vi "Adding camera trigger to counter task_final.vi"() -> ()   [LabVIEW 2020]
uses:
  <vilib>/DAQmx/write.llb/DAQmx Write (Analog 1D DBL 1Chan NSamp).vi
  <vilib>/DAQmx/create/channels.llb/DAQmx Create Channel (AO-Voltage-Basic).vi
  <vilib>/Analysis/polynomials.llb/Polynomial Plot (Range).vi
  <vilib>/Utility/file.llb/Read Delimited Spreadsheet (DBL).vi
  <vilib>/DAQmx/configure/timing.llb/DAQmx Timing (Sample Clock).vi
  <vilib>/DAQmx/miscellaneous.llb/DAQmx Fill In Error Info.vi
  <vilib>/DAQmx/create/channels.llb/DAQmx Create Channel (CO-Pulse Generation-Frequency).vi
  <vilib>/DAQmx/configure/timing.llb/DAQmx Timing (Implicit).vi
  <vilib>/DAQmx/create/channels.llb/DAQmx Create Channel (CO-Pulse Generation-Ticks).vi
  <resource>/objmgr/daqmx.rc
  <vilib>/Analysis/NI_AALPro.lvlib
panel:
  in  "How many datapoints?":i32=1025
  in  "File to read":path=path "C:/Users/Hannah/Downloads/newcalibration_voice coil input_25msflyback.txt"
  in  "P(x)":dbl[](array[numeric])=[-0.285, 0.654, -0.163]
  out "polynomial plot":cluster{dbl[], "P(A)":dbl[]}(graph)
  out "# Samples written per channel":u32=1000
  out "actual frequency":dbl=1000.0
  in  "stop":bool
  out "Signal input to voice coil (blue)":dbl[](graph)
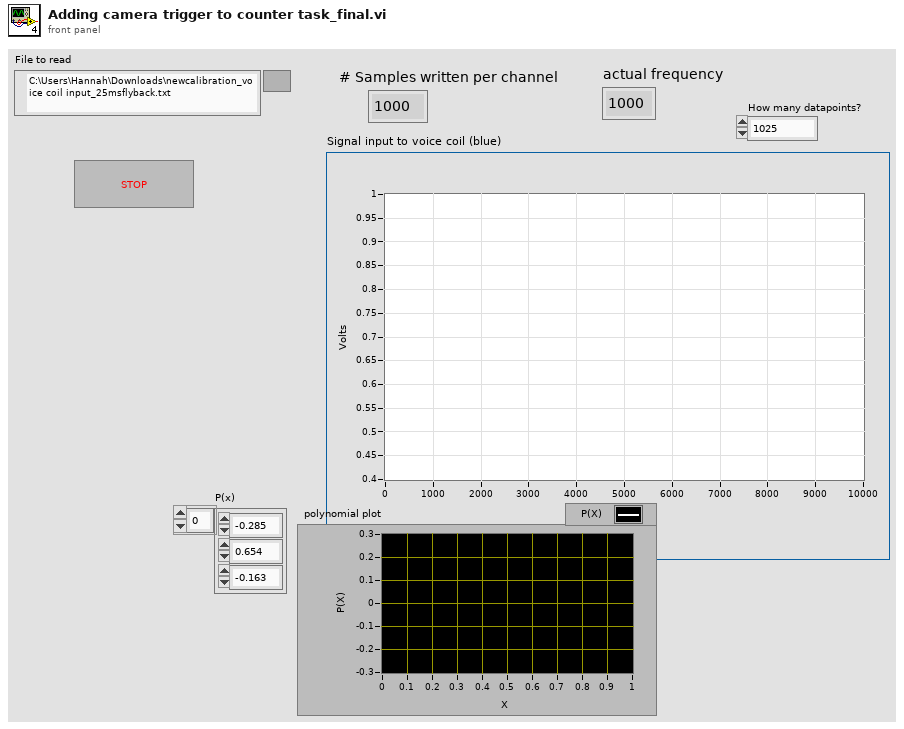
[diagram p1: front panel]
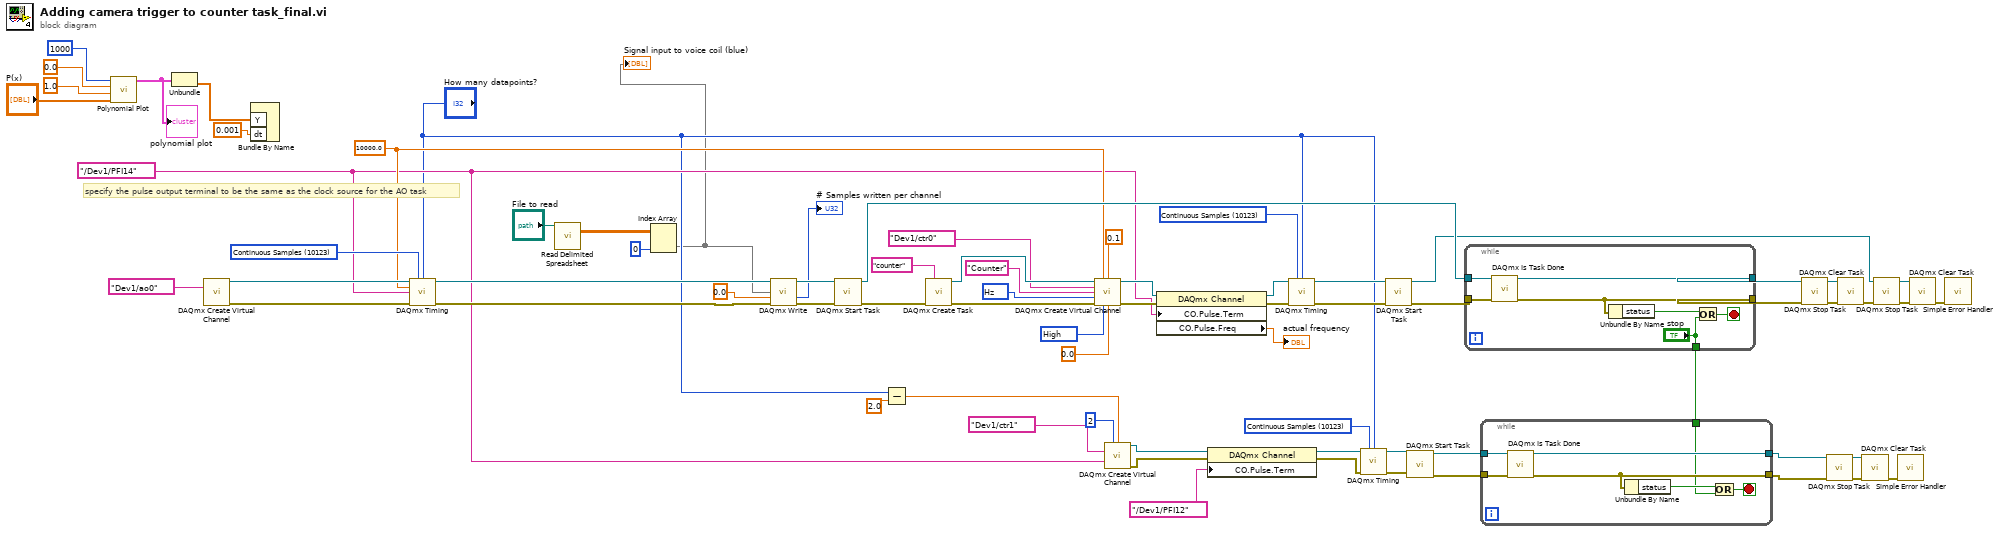
[diagram p0: block diagram]
diagram:
  w10 = 10123 items=["Finite Samples"=10178, "Continuous Samples"=10123, "Hardware Timed Single Point"=12522] ("sample mode")
  w43 = 10192 items=["High"=10192, "Low"=10214] ("idle state")
  w44 = 10373 items=["Hz"=10373] ("units")
  w7 = tag "/Dev1/PFI14" ("CO.Pulse.Term")
  w24 = 10123 items=["Finite Samples"=10178, "Continuous Samples"=10123, "Hardware Timed Single Point"=12522] ("sample mode")
  w20 = 10000.0 ("rate")
  w70 = 10123 items=["Finite Samples"=10178, "Continuous Samples"=10123, "Hardware Timed Single Point"=12522] ("sample mode")
  # "specify the pulse output terminal to be the same as the clock source for the AO task"
  n1 = call-poly <vilib>:"Polynomial Plot.vi"("P(x)"="P(x)", "end"=1.0, "start"=0.0, "samples"=1000) -> ("polynomial plot"=w38:cluster{"Ramp Pattern":dbl[], "P(A)":dbl[]})  [unwired: 6 in, 1 out]
  "polynomial plot" <- w38
  n2 = Unbundle(w38) -> ("P(A)"=w2:dbl[])  [unwired: 1 out]
  n3 = call-poly <vilib>:"DAQmx Create Virtual Channel.vi"("physical channels"=tag "Dev1/ao0") -> ("task out"=w72:refnum<k21>, "error out"=w71:errorcluster)  [unwired: 13 in]
  n4 = Bundle By Name("Y"=w2, "dt"=0.001) -> ()  [unwired: 1 in, 1 out]
  n5 = call-poly <vilib>:"DAQmx Timing.vi"("task/channels in"=w72, "sample mode"=w70, "samples per channel"="How many datapoints?", "rate"=w20, "source"=w7, "error in"=w71) -> ("task out"=w28:refnum<k21>, "error out"=w27:errorcluster)  [unwired: 8 in]
  n6 = call-poly <vilib>:"Read Delimited Spreadsheet.vi"("file path (dialog if empty)"="File to read") -> ("all rows"=w32:dbl[][])  [unwired: 9 in, 5 out]
  n7 = Index Array(array=w32, index (col)=0 ("disabled index (col)")) -> (element=w1:dbl[])  [unwired: 1 in]
  "Signal input to voice coil (blue)" <- w1
  n8 = call-poly <vilib>:"DAQmx Write.vi"("task/channels in"=w28, "data"=w1, "timeout"=0.0, "error in"=w27) -> ("task out"=w49:refnum<k21>, "number of samples written per channel"=→"# Samples written per channel":u32, "error out"=w48:errorcluster)  [unwired: 9 in]
  n9 = call <vilib>:"DAQmx Start Task.vi"("task/channels in"=w49, "error in"=w48) -> ("task out"=w42:refnum<k21>, "error out"=w41:errorcluster)  [unwired: 12 in]
  n10 = Subtract(x="How many datapoints?", y=2.0) -> (x-y=w5:dbl)
  n11 = call <vilib>:"DAQmx Create Task.vi"("new task name"="counter", "error in"=w41) -> ("task out"=w65:refnum<k21>, "error out"=w63:errorcluster)  [unwired: 12 in]
  n12 = call-poly <vilib>:"DAQmx Create Virtual Channel.vi"("task in"=w65, "frequency"=w20, "duty cycle"=0.1, "counter"=tag "Dev1/ctr0", "name to assign"="Counter", "units"=w44, "error in"=w63, "idle state"=w43, "initial delay"=0.0) -> ("task out"=w62:refnum<k21>, "error out"=w61:errorcluster)  [unwired: 5 in]
  n13 = call-poly <vilib>:"DAQmx Create Virtual Channel.vi"("high ticks"=u32 2, "low ticks"=w5, "counter"=tag "Dev1/ctr1", "source of ticks"=w7) -> ("task out"=w19:refnum<k21>, "error out"=w18:errorcluster)  [unwired: 10 in]
  n14 = property class="DAQmx Channel"(reference=w62, error in=w61, "CO.Pulse.Term"=w7) -> (reference out=w58:refnum<k21>, error out=w59:errorcluster, "CO.Pulse.Freq"=→"actual frequency":dbl)
  n15 = property class="DAQmx Channel"(reference=w19, error in=w18, "CO.Pulse.Term"=tag "/Dev1/PFI12") -> (reference out=w12:refnum<k21>, error out=w11:errorcluster)
  n16 = call-poly <vilib>:"DAQmx Timing.vi"("task/channels in"=w58, "sample mode"=w24, "samples per channel"="How many datapoints?", "error in"=w59) -> ("task out"=w68:refnum<k21>, "error out"=w67:errorcluster)  [unwired: 10 in]
  n17 = call-poly <vilib>:"DAQmx Timing.vi"("task/channels in"=w12, "sample mode"=w10, "samples per channel"="How many datapoints?", "error in"=w11) -> ("task out"=w9:refnum<k21>, "error out"=w8:errorcluster)  [unwired: 10 in]
  n18 = call <vilib>:"DAQmx Start Task.vi"("task/channels in"=w68, "error in"=w67) -> ("task out"=w30:refnum<k21>, "error out"=w50:errorcluster)  [unwired: 12 in]
  n19 = call <vilib>:"DAQmx Start Task.vi"("task/channels in"=w9, "error in"=w8) -> ("task out"=w16:refnum<k21>, "error out"=w15:errorcluster)  [unwired: 12 in]
  n20 = while {
    tunnel: w42 -> [w80]
    tunnel: w50 -> [w79]
    tunnel: [w78] -> w54
    tunnel: [w77] -> w55
    tunnel: ["stop"] -> w3
    stop <- w75 stop-if-true
    n21 = call <vilib>:"DAQmx Is Task Done.vi"("task/channels in"=w80, "error in"=w79) -> ("task out"=w78:refnum<k21>, "error out"=w77:errorcluster)  [unwired: 11 in, 1 out]
    n22 = Unbundle By Name(w77) -> ("status"=w76:bool)
    n23 = Or(x=w76, y="stop") -> (x .or. y?=w75:bool)
  }
  n24 = while {
    tunnel: w16 -> [w87]
    tunnel: w15 -> [w86]
    tunnel: [w85] -> w14
    tunnel: [w84] -> w13
    tunnel: w3 -> [w81]
    stop <- w82 stop-if-true
    n25 = call <vilib>:"DAQmx Is Task Done.vi"("task/channels in"=w87, "error in"=w86) -> ("task out"=w85:refnum<k21>, "error out"=w84:errorcluster)  [unwired: 11 in, 1 out]
    n26 = Unbundle By Name(w84) -> ("status"=w83:bool)
    n27 = Or(x=w83, y=w81) -> (x .or. y?=w82:bool)
  }
  n28 = call <vilib>:"DAQmx Stop Task.vi"("task/channels in"=w54, "error in"=w55) -> ("task out"=w53:refnum<k21>, "error out"=w52:errorcluster)  [unwired: 12 in]
  n29 = call <vilib>:"DAQmx Stop Task.vi"("task/channels in"=w14, "error in"=w13) -> ("task out"=w22:refnum<k21>, "error out"=w23:errorcluster)  [unwired: 12 in]
  n30 = call <vilib>:"DAQmx Clear Task.vi"("task in"=w53, "error in"=w52) -> ("error out"=w29:errorcluster)  [unwired: 13 in]
  n31 = call <vilib>:"DAQmx Clear Task.vi"("task in"=w22, "error in"=w23) -> ("error out"=w21:errorcluster)  [unwired: 13 in]
  n32 = call <vilib>:"DAQmx Stop Task.vi"("task/channels in"=w30, "error in"=w29) -> ("task out"=w56:refnum<k21>, "error out"=w57:errorcluster)  [unwired: 12 in]
  n33 = call <vilib>:"Simple Error Handler.vi"("error in (no error)"=w21) -> ()  [unwired: 4 in, 5 out]
  n34 = call <vilib>:"DAQmx Clear Task.vi"("task in"=w56, "error in"=w57) -> ("error out"=w51:errorcluster)  [unwired: 13 in]
  n35 = call <vilib>:"Simple Error Handler.vi"("error in (no error)"=w51) -> ()  [unwired: 4 in, 5 out]
